vi "Climber_Test.vi"(1 "Joystick_Out":T1={"Pilot Left Joystick X"=0.0, "Pilot Left Joystick Y"=-0.0, "Pilot A Button"=FALSE, "Pilot B Button"=FALSE, "Pilot X Button"=FALSE, "Pilot Y Button"=FALSE, "Pilot Left Bumper"=FALSE, "Pilot Right Bumper"=FALSE, "Pilot View Button"=FALSE, "Pilot Menu Button"=FALSE, "Pilot Left Joystick Press"=FALSE, "Pilot Right Joystick Press"=FALSE, "Pilot Left Trigger"=0.0, "Pilot Right Joystick X"=0.0, "Pilot Right Joystick Y"=0.0, "Pilot Right Trigger"=0.0, "Copilot Left Joystick X"=0.0, "Copilot Left Joystick Y"=0.0, "Copilot A Button"=FALSE, "Copilot B Button"=FALSE, "Copilot X Button"=FALSE, "Copilot Y Button"=FALSE, "Copilot Left Bumper"=FALSE, "Copilot Right Bumper"=FALSE, "Copilot View Button"=FALSE, "Copilot Menu Button"=FALSE, "Copilot Left Joystick Press"=FALSE, "Copilot Right Joystick Press"=FALSE, "Copilot Left Trigger"=0.0, "Copilot Right Joystick X"=0.0, "Copilot Right Joystick Y"=0.0, "Copilot Right Trigger"=0.0, "Pilot D-pad North"=FALSE, "Pilot D-pad South"=FALSE, "Pilot D-pad East"=FALSE, "Pilot D-pad West"=FALSE, "Pilot D-pad NE "=FALSE, "Pilot D-pad SE"=FALSE, "Pilot D-pad SW"=FALSE, "Pilot D-pad NW"=FALSE, "CoPilot D-pad North"=FALSE, "CoPilot D-pad South"=FALSE, "CoPilot D-pad East"=FALSE, "CoPilot D-pad West"=FALSE, "CoPilot D-pad NE"=FALSE, "CoPilot D-pad SE"=FALSE, "CoPilot D-pad SW"=FALSE, "CoPilot D-pad NW"=FALSE, "Pilot Left Trigger Pressed"=FALSE, "Pilot Right Trigger Pressed"=FALSE, "CoPilot Left Trigger Pressed"=FALSE, "CoPilot Right Trigger Pressed"=FALSE}) -> ()   [LabVIEW 2020]
uses:
  Utility VIs/Joystick_Controls.ctl
  Subsystems/Climber/Climber_Cluster.ctl
  Subsystems/Climber/Climber_Control_States.ctl
  Globals/Climber_Globals.vi
panel:
  in  "Inner Pivot Left Trigger Deadzone Size":dbl=0.1 format="%#_13g"
  in  "Inner Pivot Right Trigger Deadzone Size":dbl=0.1 format="%#_13g"
  in  "Outer Elevator Deadzone Size":dbl=0.1 format="%#_13g"
  in  "Outer Pivot Deadzone Size":dbl=0.1 format="%#_13g"
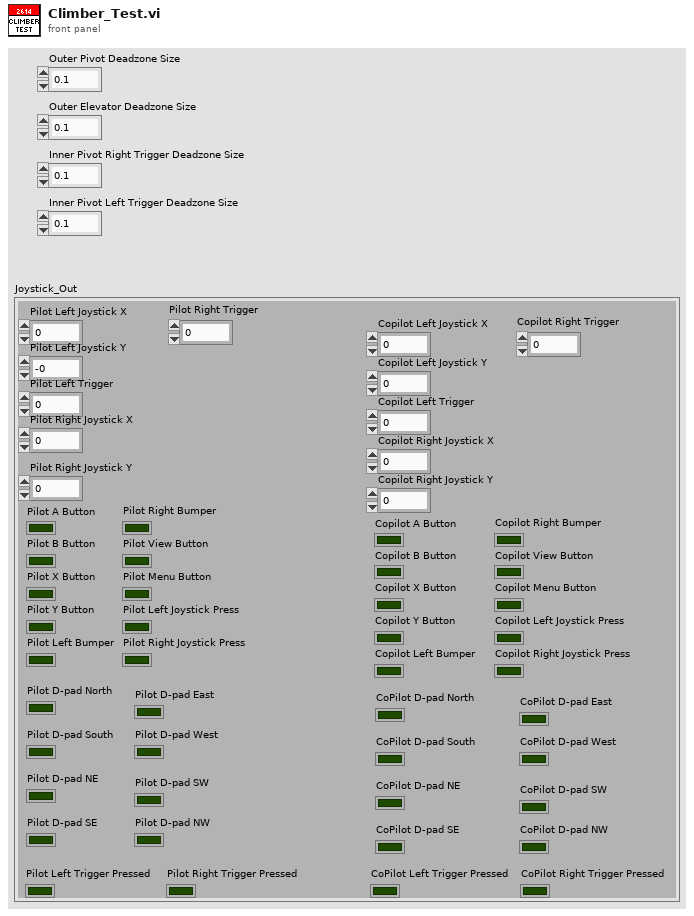
[diagram p1: front panel]
types:
  T1 = typedef "Joystick_Controls.ctl" = cluster{"Pilot Left Joystick X":dbl, "Pilot Left Joystick Y":dbl, "Pilot A Button":bool, "Pilot B Button":bool, "Pilot X Button":bool, "Pilot Y Button":bool, "Pilot Left Bumper":bool, "Pilot Right Bumper":bool, "Pilot View Button":bool, "Pilot Menu Button":bool, "Pilot Left Joystick Press":bool, "Pilot Right Joystick Press":bool, "Pilot Left Trigger":dbl, "Pilot Right Joystick X":dbl, "Pilot Right Joystick Y":dbl, "Pilot Right Trigger":dbl, "Copilot Left Joystick X":dbl, "Copilot Left Joystick Y":dbl, "Copilot A Button":bool, "Copilot B Button":bool, "Copilot X Button":bool, "Copilot Y Button":bool, "Copilot Left Bumper":bool, "Copilot Right Bumper":bool, "Copilot View Button":bool, "Copilot Menu Button":bool, "Copilot Left Joystick Press":bool, "Copilot Right Joystick Press":bool, "Copilot Left Trigger":dbl, "Copilot Right Joystick X":dbl, "Copilot Right Joystick Y":dbl, "Copilot Right Trigger":dbl, "Pilot D-pad North":bool, "Pilot D-pad South":bool, "Pilot D-pad East":bool, "Pilot D-pad West":bool, "Pilot D-pad NE ":bool, "Pilot D-pad SE":bool, "Pilot D-pad SW":bool, "Pilot D-pad NW":bool, "CoPilot D-pad North":bool, "CoPilot D-pad South":bool, "CoPilot D-pad East":bool, "CoPilot D-pad West":bool, "CoPilot D-pad NE":bool, "CoPilot D-pad SE":bool, "CoPilot D-pad SW":bool, "CoPilot D-pad NW":bool, "Pilot Left Trigger Pressed":bool, "Pilot Right Trigger Pressed":bool, "CoPilot Left Trigger Pressed":bool, "CoPilot Right Trigger Pressed":bool}
  T2 = typedef "Climber_Cluster.ctl" = cluster{"Control_State":T3, "Outer_Arm_Pivot_Throttle":dbl, "Outer_Arm_Elevator_Throttle":dbl, "Inner_Arm_Pivot_Throttle":dbl, "Enable_Climber_Sequence":bool}
  T3 = typedef "Climber_Control_States.ctl" = enum16{"No-Op", "Manual_%Vbus", "Correct_Outer_Pivot_Offset", "Climbing_Sequence"}
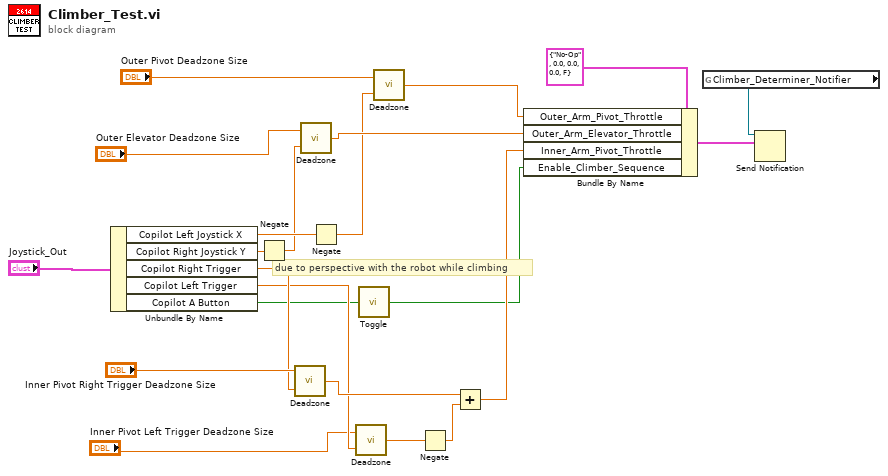
[diagram p0: block diagram]
diagram:
  # "due to perspective with the robot while climbing"
  n1 = Unbundle By Name("Joystick_Out") -> ("Copilot Left Joystick X"=w15:dbl, "Copilot Right Joystick Y"=w4:dbl, "Copilot Right Trigger"=w11:dbl, "Copilot Left Trigger"=w9:dbl, "Copilot A Button"=w2:bool)
  n2 = Negate(x=w4) -> (-x=w3:dbl)
  n3 = call "Deadzone.vi"("Joystick Value Input"=w11, "Deadzone Size"="Inner Pivot Right Trigger Deadzone Size") -> ("Corrected Joystick Value"=w10:dbl)  [unwired: 1 in]
  n4 = call "Deadzone.vi"("Joystick Value Input"=w3, "Deadzone Size"="Outer Elevator Deadzone Size") -> ("Corrected Joystick Value"=w6:dbl)  [unwired: 1 in]
  n5 = Negate(x=w15) -> (-x=w5:dbl)
  n6 = call "Deadzone.vi"("Joystick Value Input"=w9, "Deadzone Size"="Inner Pivot Left Trigger Deadzone Size") -> ("Corrected Joystick Value"=w7:dbl)  [unwired: 1 in]
  n7 = call "Toggle.vi"("Boolean"=w2) -> ("Boolean Out"=w1:bool)
  n8 = call "Deadzone.vi"("Joystick Value Input"=w5, "Deadzone Size"="Outer Pivot Deadzone Size") -> ("Corrected Joystick Value"=w14:dbl)  [unwired: 1 in]
  n9 = Negate(x=w7) -> (-x=w17:dbl)
  n10 = Add(x=w10, y=w17) -> (x+y=w20:dbl)
  n11 = Bundle By Name(cluster=T2 {"Control_State"=enum."No-Op", "Outer_Arm_Pivot_Throttle"=0.0, "Outer_Arm_Elevator_Throttle"=0.0, "Inner_Arm_Pivot_Throttle"=0.0, "Enable_Climber_Sequence"=FALSE} ("Climber_Cluster"), "Outer_Arm_Pivot_Throttle"=w14, "Outer_Arm_Elevator_Throttle"=w6, "Inner_Arm_Pivot_Throttle"=w20, "Enable_Climber_Sequence"=w1) -> (w21:T2)
  n12 = global read "Climber_Globals.vi" "Climber_Determiner_Notifier"() -> (w22:refnum<notifier>)
  n13 = Send Notification(notification=w21, notifier=w22) -> ()  [unwired: 1 in, 2 out]
